vi "RSZVB Set Port Impedances Renormalization.vi"(8 "error in (no error)":errorcluster {"code" format="%.0x"}, 9 "Theory (0: Travelling Waves)":i32(ring) items=["Travelling Waves", "Power Waves"], 10 "Channel (1)":i32=1, 11 "VISA session":refnum<visa-resource-name>) -> (0 "error out":errorcluster {"code" format="%.0x"}, 3 "dup VISA session":refnum<visa-resource-name>)   [LabVIEW 2011]
doc: "This VI selects the theory for the renormalization of port impedances. The selection has an impact on the conversion formulas for wave quantities and S-parameters.\n\nRemote-control command(s):\nCALCulate<Chn>:TRANsform:IMPedance:RNORmal TWAVes | PWAVes"
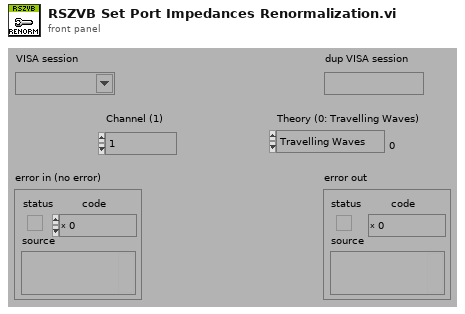
[diagram p1: front panel]
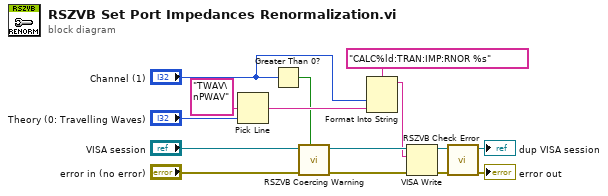
[diagram p0: block diagram]
diagram:
  n1 = Pick Line(multi-line string="TWAV\nPWAV", line index="Theory (0: Travelling Waves)") -> (output string=w12:string)  [unwired: 1 in]
  n2 = Greater Than 0?(x="Channel (1)") -> (x > 0?=w7:bool)
  n3 = call "RSZVB Coercing Warning.vi"("In Range?"=w7, "error in (no error)"="error in (no error)", "VISA session"="VISA session") -> ("error out"=w8:errorcluster, "dup VISA session"=w6:refnum<visa-resource-name>)  [unwired: 7 in]
  n4 = Format Into String(format string="CALC%ld:TRAN:IMP:RNOR %s", "Channel (1)", w12) -> (resulting string=w1:string)  [unwired: 2 in, 1 out]
  n5 = VISA Write(VISA resource name=w6, write buffer=w1, error in (no error)=w8) -> (VISA resource name out=w5:refnum<visa-resource-name>, error out=w4:errorcluster)  [unwired: 1 out]
  n6 = call "RSZVB Check Error.vi"("error in (no error)"=w4, "VISA session"=w5) -> ("error out"=→"error out":errorcluster, "dup VISA session"=→"dup VISA session":refnum<visa-resource-name>)  [unwired: 8 in]
